vi "Unwrap.vi"(11 "Channel Message":refnum<class "Channel Message.lvclass">) -> (3 "gesture":refnum<class "Gesture.lvclass">)   [LabVIEW 2019, in "Gesture Wrapper.lvclass"]
doc: "Retrieve the gesture from the Channel Message."
uses:
  Gesture Wrapper.lvclass
  Gesture/Gesture.lvclass
  <vilib>/ChannelSupport/Channel Message/Channel Message.lvclass
  Gesture Wrapper.lvclass/Gesture Wrapper.ctl
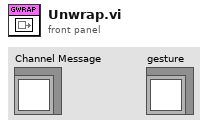
[diagram p1: front panel]
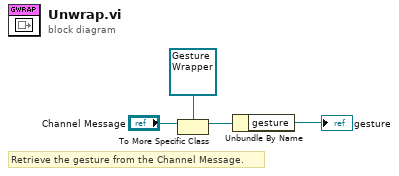
[diagram p0: block diagram]
diagram:
  # "Retrieve the gesture from the Channel Message."
  n1 = To More Specific Class(target class=refnum<class "Gesture Wrapper.lvclass"> refnum ("Gesture Wrapper"), reference="Channel Message") -> (specific class reference=w2:refnum<class "Gesture Wrapper.lvclass">)  [unwired: 1 in, 1 out]
  n2 = Unbundle By Name(w2) -> ("gesture"=→"gesture":refnum<class "Gesture.lvclass">)
